vi "JKI_ErrorHandler.vi"() -> ()   [LabVIEW 2017, in "Error Handler_JKI.lvlib"]
uses:
  APIs/Error Handler_JKI.lvlib
  <userlib>/_NEVSTOP/JKI State Machine ++/_Support/_JKISMQFGV.vi
  <userlib>/_NEVSTOP/JKI State Machine ++/JKI-State-Machine-Plus.lvlib
panel:
  in  "Error Simulator":bool
  in  "Stop Button":bool
  out "State History":string
  in  "Name(\"\" to use uuid)":string="Event JKISM"
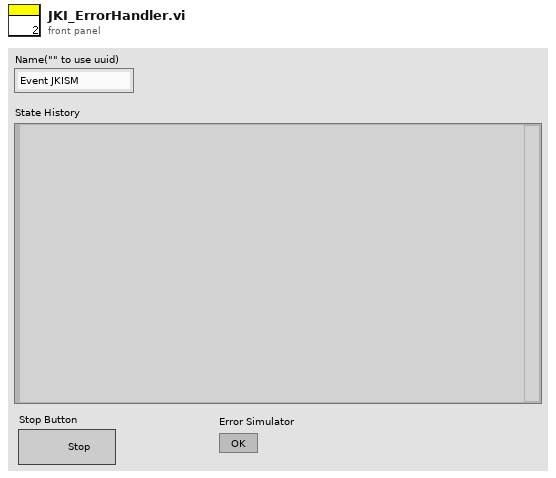
[diagram p1: front panel]
types:
  T1 = enum32{"Invalid", "Standard", "Closed", "Hidden", "Minimized", "Maximized"}
  T2 = enum32{"invalid app kind", "Development System", "Run Time System", "Student Edition", "Embedded LabVIEW", "Evaluation", "Custom"}
  T3 = enum16{"open", "replace", "create", "open or create", "replace or create", "replace or create with confirmation"}
  T4 = cluster{"Core":cluster{"Current VI Reference":refnum<vi>, "Close Panel on Exit?":bool}, "Your Boolean data":bool, "Your string data":string}
  T5 = cluster{"Current VI Reference":refnum<vi>, "Close Panel on Exit?":bool}
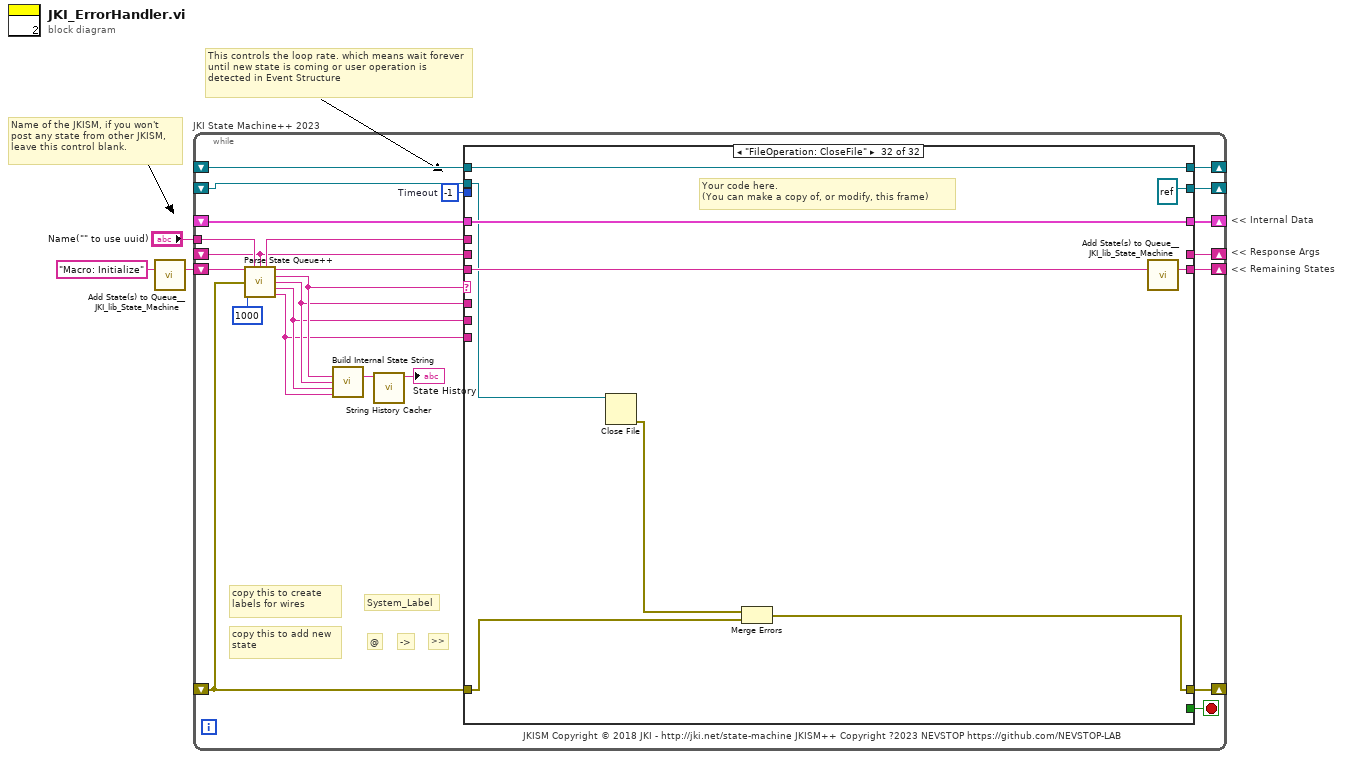
[diagram p0: block diagram]
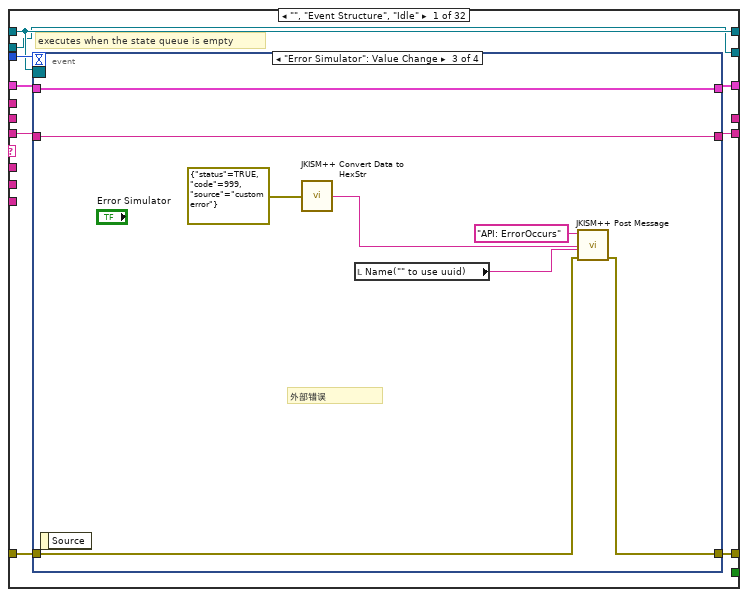
[diagram p2: hidden frame]
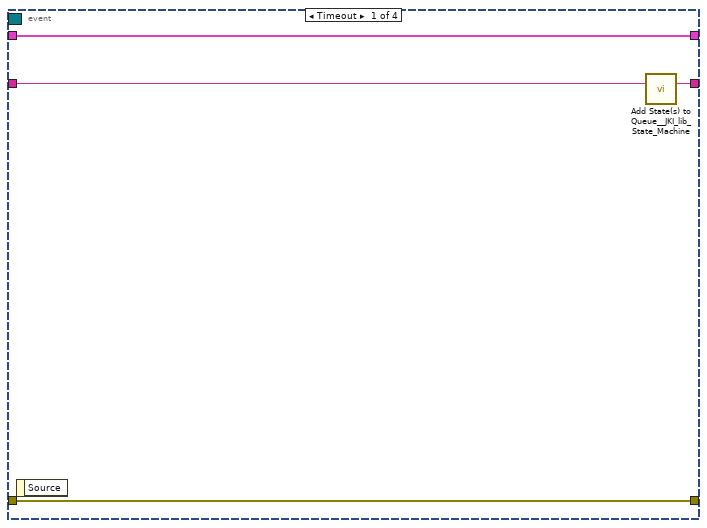
[diagram p3: hidden frame]
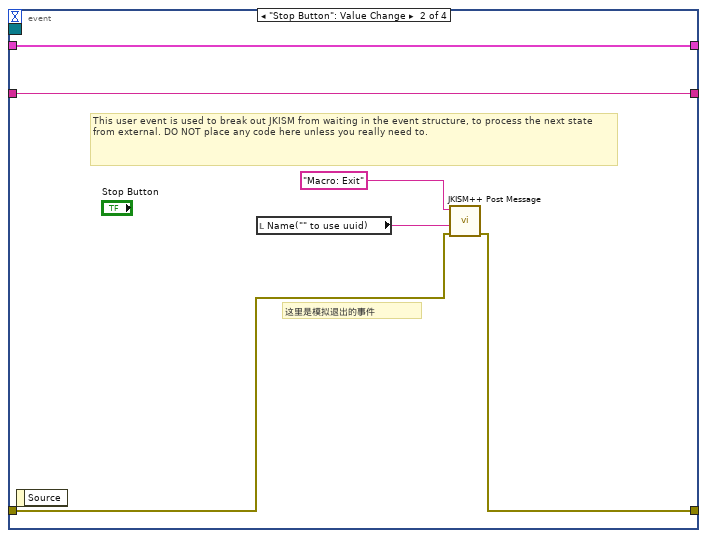
[diagram p4: hidden frame]
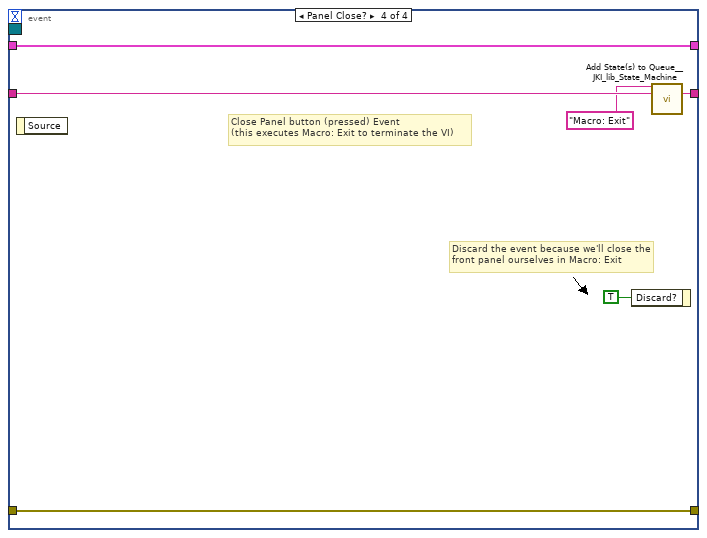
[diagram p5: hidden frame]
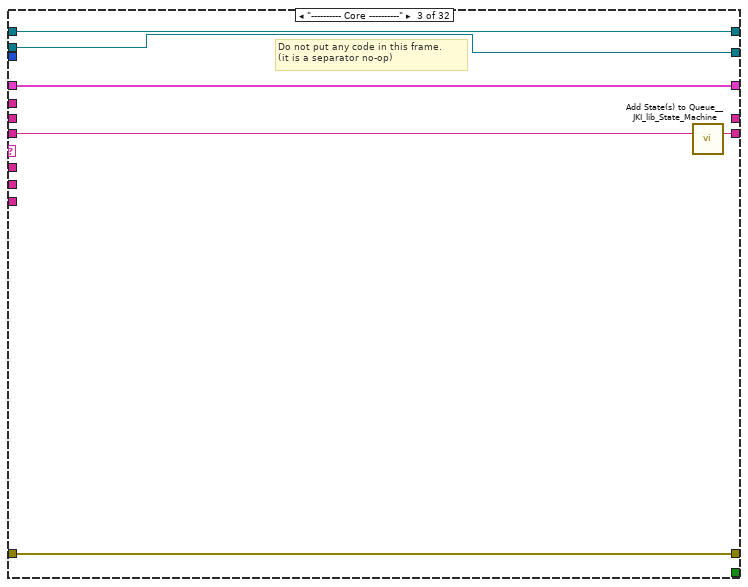
[diagram p7: hidden frame]
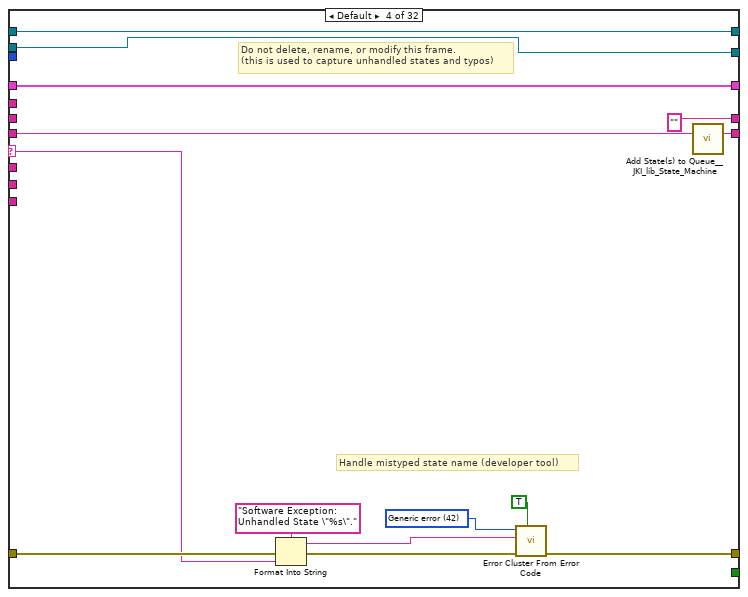
[diagram p8: hidden frame]
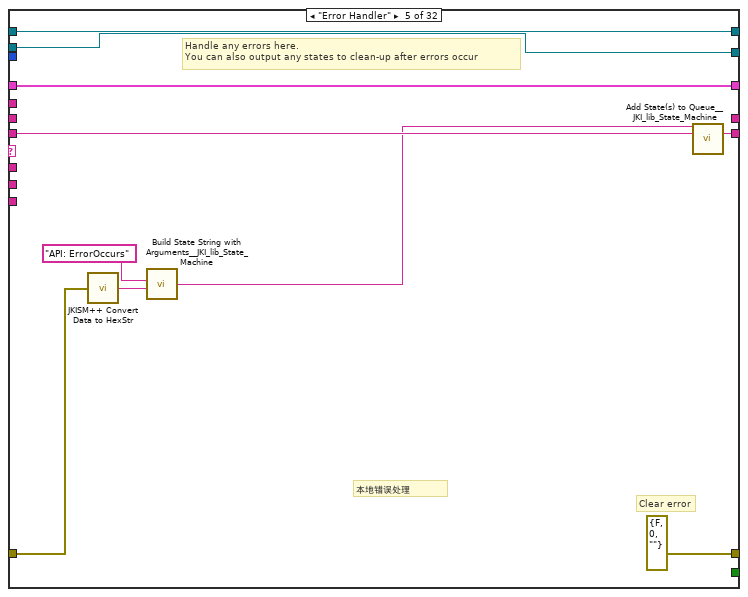
[diagram p9: hidden frame]
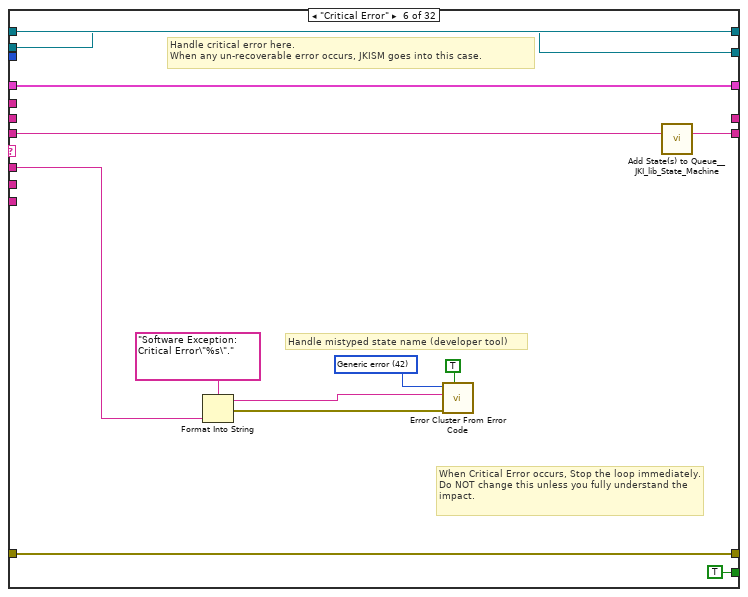
[diagram p10: hidden frame]
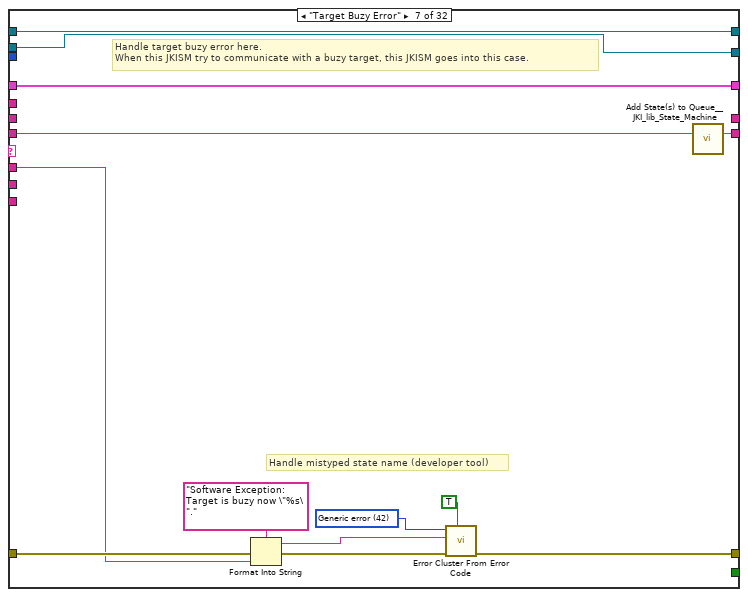
[diagram p11: hidden frame]
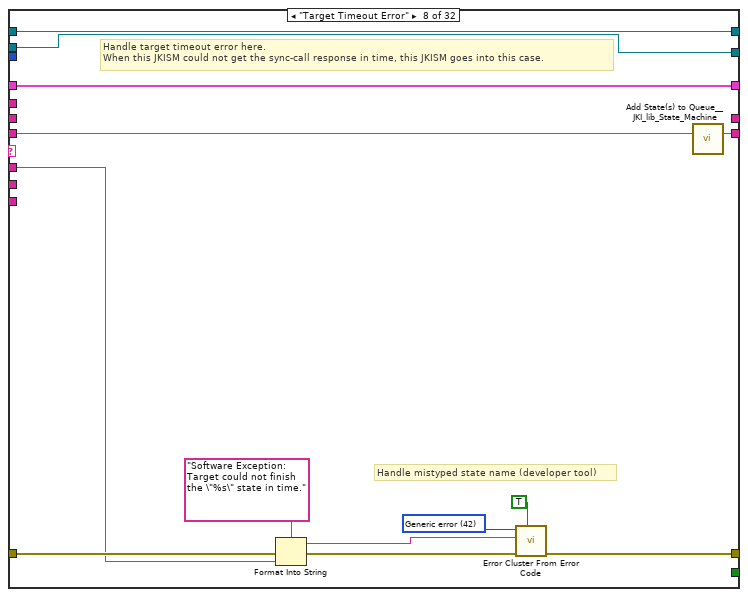
[diagram p12: hidden frame]
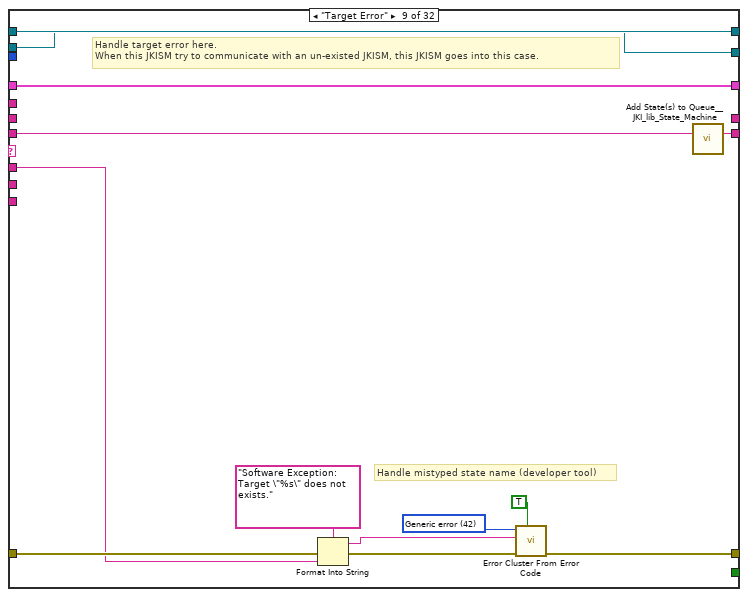
[diagram p13: hidden frame]
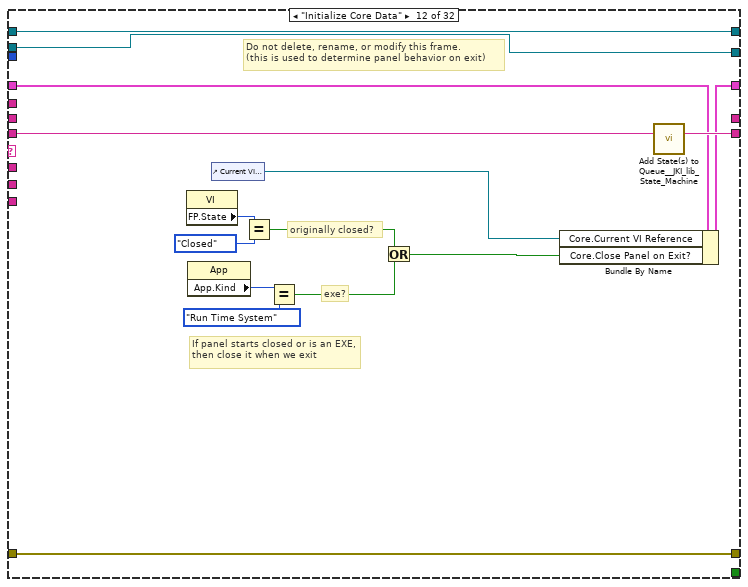
[diagram p16: hidden frame]
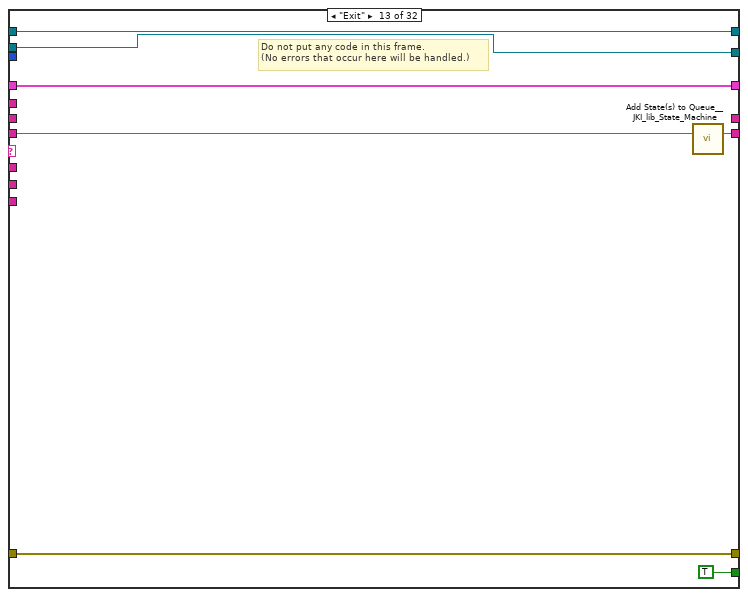
[diagram p17: hidden frame]
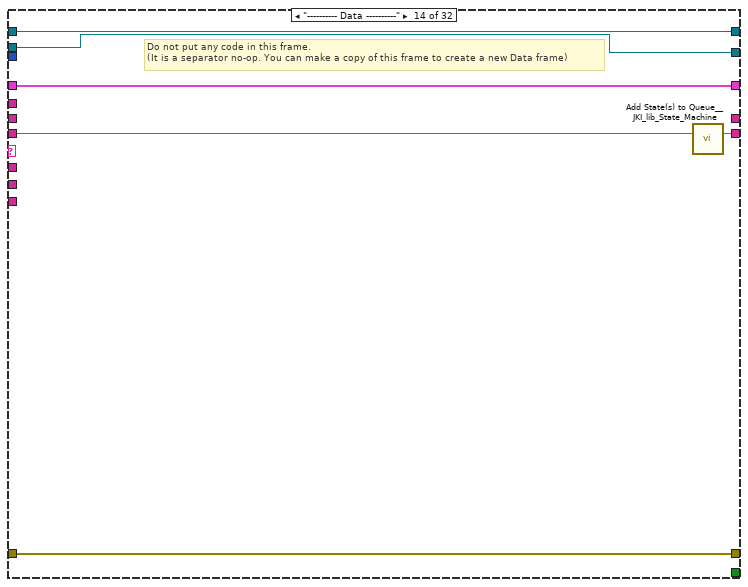
[diagram p18: hidden frame]
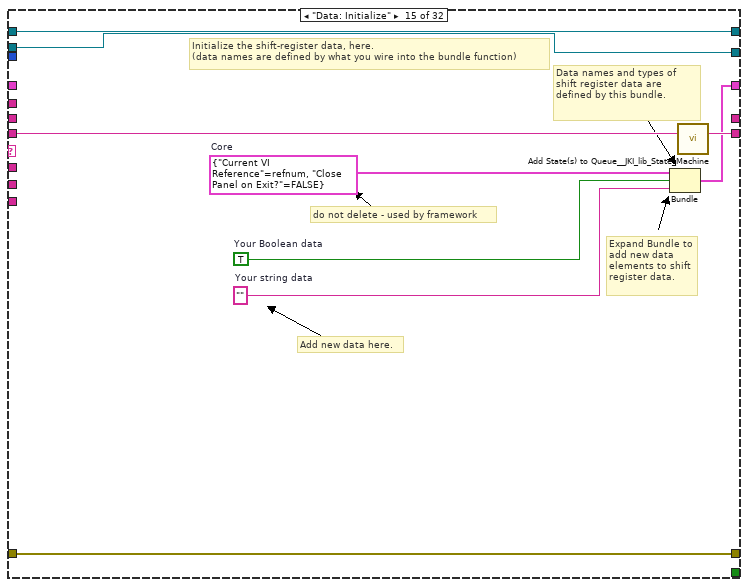
[diagram p19: hidden frame]
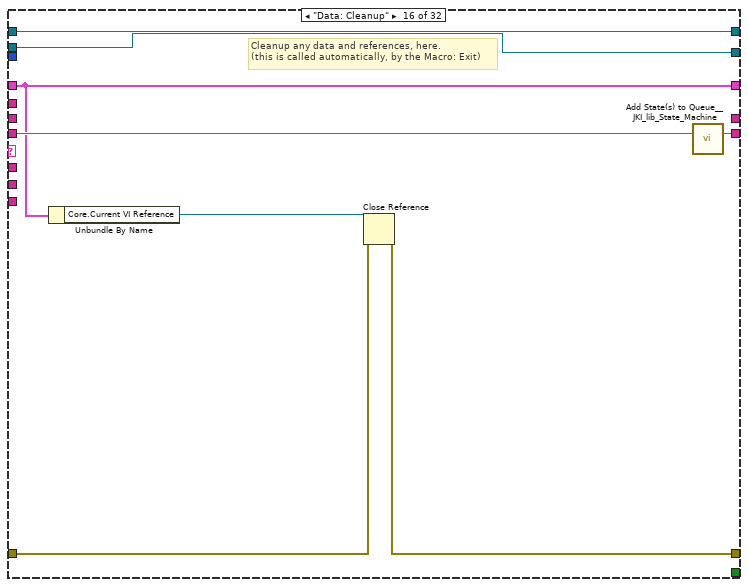
[diagram p20: hidden frame]
diagram:
  # "<< Internal Data"
  # "<< Response Args"
  # "<< Remaining States"
  # "Name of the JKISM, if you won't post any state from other JKISM,  leave this control blank."
  # "This controls the loop rate. which means wait forever until new state is coming or user operation is detected in Event Structure"
  n1 = call <vilib>:"Add State(s) to Queue__JKI_lib_State_Machine.vi"("State(s) in (\"\")"="Macro: Initialize") -> ("States Out"=w1:string)  [unwired: 14 in]
  n2 = while "JKI State Machine++ 2023" {
    shift-right: [w22] -> _
    shift-left: _ -> [w21]
    shift-right: [w25] -> _
    shift-left: _ -> [w19]
    shift-right: [w24] -> _
    shift-left: w1 -> [w26]
    tunnel: "Name(\"\" to use uuid)" -> [w14]
    shift-right: [w17] -> _
    shift-left: _ -> [w6]
    shift-right: [w16] -> _
    shift-left: _ -> [w15]
    shift-right: [w5] -> _
    shift-left: _ -> [w4]
    stop <- w23 stop-if-true
    w20 = -1  # Timeout
    # "JKISM Copyright © 2018 JKI - http://jki.net/state-machine JKISM++ Copyright ?2023 NEVSTOP https://github.com/NEVSTOP-LAB"
    # "copy this to add new state"
    # ">>"
    # "->"
    # "@"
    # "copy this to create labels for wires"
    # "System_Label"
    n3 = call <userlib>:"Parse State Queue++.vi"("State Queue"=w26, "Name(\"\" to use uuid)"=w14, "Response Arguments"=w6, "Error In (no error)"=w19, "Response Timeout(5000ms)"=1000 ("Response Timeout(1000ms)")) -> ("Name Used"=w7:string, "Remaining States"=w27:string, "Current State"=w11:string, "Arguments"=w10:string, "Argument - State"=w9:string, "From Who"=w8:string)  [unwired: 5 in]
    n4 = call <userlib>:"Build Internal State String.vi"("State"=w11, "Arguments (\"\")"=w10, "Arg-State (\"\")"=w9, "Source (\"\")"=w8) -> ("State with Arguments"=w12:string)  [unwired: 11 in]
    n5 = call <userlib>:"String History Cacher.vi"("String"=w12) -> ("String Cache"=→"State History":string)  [unwired: 10 in]
    n6 = case shown="\"FileOperation: CloseFile\"" w11 {
      selector: w11 -> [_ _ _ w75 _ _ _ _ _ _ _ _ _ _ _ _ _ _ _ _ _ _ _ _ _ _ _ _ _ _ _ _]
      tunnel: w27 -> [w36 w64 w71 w79 w95 w106 w110 w128 w141 w151 w156 w172 w179 w185 w194 w202 w208 w215 w220 w227 w233 w241 w254 w325 w332 w344 w348 w352 w374 w391 w400 w409]
      tunnel: w10 -> [_ _ _ _ _ w99 w112 w124 w137 _ _ _ _ _ _ _ _ _ _ _ _ w236 w248 _ _ _ _ w369 _ _ _ _]
      tunnel: w21 -> [w34 w63 w68 w77 w92 w107 w114 w126 w139 w150 w155 w165 w177 w182 _ w197 w205 w214 w219 w224 w231 w239 w250 w322 w329 w341 w347 w371 w380 w388 w398 w407]
      tunnel: [w33 w65 w69 w81 errorcluster {"status"=FALSE, "code"=0, "source"=""} ("error out") w108 w117 w130 w143 w152 w157 w169 w176 w183 w191 w198 w206 w210 w218 w225 w230 w237 w251 w323 w330 w342 w349 w354 w376 w389 w392 w401] -> w25
      tunnel: w19 -> [w32 w65 w69 w80 w89 w108 w116 w129 w142 w152 w157 w169 w176 w183 w191 w199 w206 _ w221 w225 w230 w238 w252 w323 w330 w342 w349 w366 w377 w389 w393 w403]
      tunnel: [w35 w64 w70 w78 w94 w105 w115 w127 w140 w151 w156 w171 w178 w184 w193 w201 w207 w215 w220 w226 w232 w240 w253 w324 w331 w343 w348 w351 w373 w390 w399 w408] -> w24
      tunnel: [_ _ _ _ _ TRUE _ _ _ _ _ _ TRUE _ _ _ _ _ _ _ _ _ _ _ _ _ _ _ TRUE _ _ _] -> w23
      tunnel: [w31 w63 w68 w77 w92 w107 w114 w126 w139 w150 w155 w170 w177 w182 w192 w197 w205 w214 w219 w224 w231 w239 w250 w322 w329 w341 w347 w371 w380 w388 w398 w407] -> w22
      tunnel: w20 -> [w30 _ _ _ _ _ _ _ _ _ _ _ _ _ _ _ _ _ _ _ _ _ _ _ _ _ _ _ _ _ _ _]
      tunnel: w8 -> [_ _ _ _ _ _ _ _ _ _ _ _ _ _ _ _ _ _ _ _ _ _ _ _ _ _ _ w362 _ _ _ _]
      tunnel: w9 -> [_ _ _ _ _ _ _ _ _ _ _ _ _ _ _ _ _ _ _ _ _ _ _ _ _ _ _ _ _ _ _ _]
      tunnel: [_ _ _ "" _ _ _ _ _ _ _ _ _ _ _ _ _ _ _ _ _ _ _ _ _ _ _ _ _ _ _ _] -> w17
      tunnel: [w29 w62 w67 w73 w91 w97 w111 w123 w136 w149 w154 w159 w174 w181 w187 w196 w204 w213 w217 w223 w229 w235 w247 w321 w327 w334 w346 w370 w379 w387 w397 w406] -> w16
      tunnel: w15 -> [w29 w62 w67 w73 w91 w97 w111 w123 w136 w149 w154 w159 w174 w181 w187 w196 w204 _ w217 w223 w229 w235 w247 w321 w327 w334 w346 w370 w379 w387 w397 w406]
      tunnel: w7 -> [_ _ _ _ _ _ _ _ _ _ _ _ _ _ _ _ _ w212 _ _ _ _ _ _ _ _ _ _ _ _ _ _]
      tunnel: w6 -> [_ _ _ _ _ _ _ _ _ _ _ _ _ _ _ _ _ _ _ _ _ _ _ _ _ _ _ _ _ _ _ _]
      tunnel: [w28 w61 w66 w72 w90 w96 w109 w122 w135 w148 w153 w158 w173 w180 w186 w195 w203 w209 w216 w222 w228 w234 w246 w320 w326 w333 w345 w353 w378 w386 w394 refnum<file> refnum ("refnum out")] -> w5
      tunnel: w4 -> [w28 w61 w66 w72 w90 w96 w109 w122 w135 w148 w153 w158 w173 w180 w186 w195 w203 w209 w216 w222 w228 w234 w246 w320 w326 w333 w345 w357 w378 w386 _ w405]
      frame "", "Event Structure", "Idle" {
        # "executes when the state queue is empty"
        n7 = event shown="[2] \"Error Simulator\": Value Change" {
          selector: w29 -> [_ _ _ _]
          dyn-events: _ -> [_ _ _ _]
          timeout: w30 -> [_ _ _ _]
          tunnel: w36 -> [w40 w45 w54 w60]
          tunnel: [w39 w45 w54 w59] -> w35
          tunnel: w34 -> [w37 w46 w53 w57]
          tunnel: [w38 w41 w47 w58] -> w33
          tunnel: w32 -> [w38 w42 w48 w58]
          tunnel: [w37 w46 w53 w57] -> w31
          event Timeout {
            n8 = event-data() -> ()  [unwired: 1 in, 1 out]
            n9 = call <vilib>:"Add State(s) to Queue__JKI_lib_State_Machine.vi"("State(s) in (\"\")"=w40) -> ("States Out"=w39:string)  [unwired: 14 in]
          }
          event "Stop Button": Value Change {
            # "这里是模拟退出的事件"
            # "This user event is used to break out JKISM from waiting in the event structure, to process the next state from external. DO NOT place any code here unless you really need to."
            n10 = event-data() -> ()  [unwired: 1 in, 1 out]
            n11 = local read "Name(\"\" to use uuid)"() -> (w44:string)
            n12 = call <userlib>:"JKISM++ Post Message.vi"("Error In (no error)"=w42, "Dest Module"=w44, "States"="Macro: Exit" ("Name(\"\" to use uuid)")) -> ("error IO"=w41:errorcluster)  [unwired: 8 in]
          }
          event "Error Simulator": Value Change {
            # "外部错误"
            n13 = event-data() -> ()  [unwired: 1 in, 1 out]
            n14 = call <userlib>:"JKISM++ Convert Data to HexStr.vi"("Variant"=errorcluster {"status"=TRUE, "code"=999, "source"="custom error"} ("error in (no error)")) -> ("HEX String (0-9,A-F)"=w49:string)  [unwired: 8 in]
            n15 = local read "Name(\"\" to use uuid)"() -> (w52:string)
            n16 = call <userlib>:"JKISM++ Post Message.vi"("Error In (no error)"=w48, "Dest Module"=w52, "Arguments (\"\")"=w49, "States"="API: ErrorOccurs") -> ("error IO"=w47:errorcluster)  [unwired: 7 in]
          }
          event Panel Close? {
            # "Discard the event because we'll close the front panel ourselves in Macro: Exit"
            # "Close Panel button (pressed) Event\n(this executes Macro: Exit to terminate the VI)"
            n17 = event-data() -> ()  [unwired: 1 in, 1 out]
            n18 = event-data("Discard?"=TRUE) -> ()  [unwired: 1 in, 1 out]
            n19 = call <vilib>:"Add State(s) to Queue__JKI_lib_State_Machine.vi"("State(s) in Front (\"\")"="Macro: Exit", "State(s) in (\"\")"=w60) -> ("States Out"=w59:string)  [unwired: 13 in]
          }
        }
      }
      frame "JKISM++ Documentation" {
        # "JKISM++ Documentation"
        # "State Syntax:\nStateCategory: State >> Argument @|-> JKISMName\nLine Terminator: Line feed\n\nExample:\nUI: Help >> About @Main\nUI: Help >> About ->Main"
        # "Commenting:\nTo add a comment use \"//\" or \"#\" and all text to the right will be ignored\nCommenting Example:\nUI: Initialize // This initializes the UI\n# This whole line is a comment\n// Another comment line"
        # "Where \"UI\" is the state category\nWhere \"Help\" is the state\nWhere \"About\" is the argument\nWhere \"Main\" is the Name of JKISM,which actually run the \"UI: Help >> About\"\n\n    \"@\" stands for sync state. Current JKISM will wait until the state is finished. \n            - if \"Main\" named JKISM does not exist, \"Target Error\" will occur.\n            - if \"Main\" named JKISM is in another sync remote state, \"Target Buzy Error\" will occur.\n            - if \"Main\" named JKISM could not finish the state in time, \"Target Timeout Error\" will occur.\n            - if everything is right. \"Response\" will occur with Argument back from \"Main\" named JKISM. \n\n    \"->\" stands for async state. Current JKISM will post the state and continue to next state in next iteration.\n            - if \"Main\" named JKISM does not exist, \"Target Error\" will occur.\n            - if everything is right. \"Async Message Posted\" will occur.\n            - After State is finished. Caller will receive a \"Async Response\" state from callee.\n\nWhen duplicated name is used for multiple JKISM module or some framework problem happens, \"Critical Error\" will occur."
      }
      frame "---------- Core ----------" {
        # "Do not put any code in this frame.\n(it is a separator no-op)"
        n20 = call <vilib>:"Add State(s) to Queue__JKI_lib_State_Machine.vi"("State(s) in (\"\")"=w71) -> ("States Out"=w70:string)  [unwired: 14 in]
      }
      frame Default {
        w84 = 42 items=["No error", "Argument error", "Memory is full", "Out of zone", "End of file", "File already open", "Generic file I/O error", "File not found", "File permission error", "Disk is full", "Duplicate path", "Too many files open", "System feature not enabled", "Resource file not found", "Cannot add resource", "Resource not found", "Image not found", "Image memory error", "Pen does not exist", "Config type invalid", "Config token not found", "Config parse error", "Config memory error", "Bad external code format", "Bad external code offset", "External code not present", "Null window", "Destroy window error", "Null menu", "Print aborted", "Bad print record", "Print driver error", "Windows error during printing", "Memory error during printing", "Print dialog error", "Generic print error", "Invalid device refnum", "Device not found", "Device parameter error", "Device unit error", "Cannot open device", "Device call aborted", "Generic error", "Cancelled by user", "Object ID too low", "Object ID too high", "Object not in heap", "Unknown heap", "Unknown object (invalid DefProc)", "Unknown object (DefProc not in table)", "Message out of range", "Invalid (null) method", "Unknown message", "Manager call not supported", "Bad address", "Network operation in progress", "Network operation timed out", "Connection is busy", "Network attribute not supported", "Network error", "Address in use", "System out of memory", "Connection aborted", "Connection refused", "Not connected", "Already connected", "Connection closed", "Initialization error (interapplication manager)", "Bad occurrence", "Wait on unbound occurrence handler", "Occurrence queue overflow", "Datalog type conflict", "Unused", "Unrecognized type (interapplication manager)", "Memory corrupt", "Failed to make temporary DLL", "Old CIN version", "Drag socket not found", "Failed to load drop-object", "Failed to register OLE object", "Failed to release OLE object", "Format specifier type mismatch", "Unknown format specifier", "Too few format specifiers", "Too many format specifiers", "Scan failed", "Newer CIN version", "Error converting to variant", "Runtime menu error", "Password tampered", "Variant attribute not found", "Incompatible variant data type", "Event data is not available", "Event Store is not present", "Occurrence is not found", "Event Queue is not created", "Event info is not available", "Refnum passed is NULL", "Error retrieving Class GUID", "Error retrieving CoClass GUID", "Error retrieving TypeLib GUID.", "Bad built application magic bytes.", "Specific driver is different from the specific driver associated with the Logical Name.", "There is no session opened to the class driver.", "Max Error", "MAX - Error with config objects", "MAX - Error loading configuration", "MAX - Group not supported"]
        # "Do not delete, rename, or modify this frame.\n(this is used to capture unhandled states and typos)"
        # "Handle mistyped state name (developer tool)"
        n21 = Format Into String(format string="Software Exception: Unhandled State \"%s\"." ("message"), error in=w80, w75) -> (resulting string=w83:string, error out=w82:errorcluster)  [unwired: 1 in]
        n22 = call <vilib>:"Error Cluster From Error Code.vi"("show call chain? (False)"=TRUE, "error in (no error)"=w82, "error message (\"\")"=w83, "error code (0)"=w84) -> ("error out"=w81:errorcluster)  [unwired: 5 in]
        n23 = call <vilib>:"Add State(s) to Queue__JKI_lib_State_Machine.vi"("State(s) in (\"\")"=w79) -> ("States Out"=w78:string)  [unwired: 14 in]
      }
      frame "Error Handler" {
        # "本地错误处理"
        # "Handle any errors here.\nYou can also output any states to clean-up after errors occur"
        # "Clear error"
        n24 = call <userlib>:"JKISM++ Convert Data to HexStr.vi"("Variant"=w89) -> ("HEX String (0-9,A-F)"=w88:string)  [unwired: 8 in]
        n25 = call <vilib>:"Build State String with Arguments__JKI_lib_State_Machine.vi"("Arguments (\"\")"=w88, "State"="API: ErrorOccurs") -> ("State with Arguments"=w86:string)  [unwired: 4 in]
        n26 = call <vilib>:"Add State(s) to Queue__JKI_lib_State_Machine.vi"("State(s) in Front (\"\")"=w86, "State(s) in (\"\")"=w95) -> ("States Out"=w94:string)  [unwired: 13 in]
      }
      frame "Critical Error" {
        w103 = 42 items=["No error", "Argument error", "Memory is full", "Out of zone", "End of file", "File already open", "Generic file I/O error", "File not found", "File permission error", "Disk is full", "Duplicate path", "Too many files open", "System feature not enabled", "Resource file not found", "Cannot add resource", "Resource not found", "Image not found", "Image memory error", "Pen does not exist", "Config type invalid", "Config token not found", "Config parse error", "Config memory error", "Bad external code format", "Bad external code offset", "External code not present", "Null window", "Destroy window error", "Null menu", "Print aborted", "Bad print record", "Print driver error", "Windows error during printing", "Memory error during printing", "Print dialog error", "Generic print error", "Invalid device refnum", "Device not found", "Device parameter error", "Device unit error", "Cannot open device", "Device call aborted", "Generic error", "Cancelled by user", "Object ID too low", "Object ID too high", "Object not in heap", "Unknown heap", "Unknown object (invalid DefProc)", "Unknown object (DefProc not in table)", "Message out of range", "Invalid (null) method", "Unknown message", "Manager call not supported", "Bad address", "Network operation in progress", "Network operation timed out", "Connection is busy", "Network attribute not supported", "Network error", "Address in use", "System out of memory", "Connection aborted", "Connection refused", "Not connected", "Already connected", "Connection closed", "Initialization error (interapplication manager)", "Bad occurrence", "Wait on unbound occurrence handler", "Occurrence queue overflow", "Datalog type conflict", "Unused", "Unrecognized type (interapplication manager)", "Memory corrupt", "Failed to make temporary DLL", "Old CIN version", "Drag socket not found", "Failed to load drop-object", "Failed to register OLE object", "Failed to release OLE object", "Format specifier type mismatch", "Unknown format specifier", "Too few format specifiers", "Too many format specifiers", "Scan failed", "Newer CIN version", "Error converting to variant", "Runtime menu error", "Password tampered", "Variant attribute not found", "Incompatible variant data type", "Event data is not available", "Event Store is not present", "Occurrence is not found", "Event Queue is not created", "Event info is not available", "Refnum passed is NULL", "Error retrieving Class GUID", "Error retrieving CoClass GUID", "Error retrieving TypeLib GUID.", "Bad built application magic bytes.", "Specific driver is different from the specific driver associated with the Logical Name.", "There is no session opened to the class driver.", "Max Error", "MAX - Error with config objects", "MAX - Error loading configuration", "MAX - Group not supported"]
        # "Handle critical error here.\nWhen any un-recoverable error occurs, JKISM goes into this case."
        # "When Critical Error occurs, Stop the loop immediately. Do NOT change this unless you fully understand the impact."
        # "Handle mistyped state name (developer tool)"
        n27 = Format Into String(format string="Software Exception: Critical Error\"%s\"." ("message"), w99) -> (resulting string=w102:string, error out=w101:errorcluster)  [unwired: 2 in]
        n28 = call <vilib>:"Error Cluster From Error Code.vi"("show call chain? (False)"=TRUE, "error in (no error)"=w101, "error message (\"\")"=w102, "error code (0)"=w103) -> ()  [unwired: 5 in, 1 out]
        n29 = call <vilib>:"Add State(s) to Queue__JKI_lib_State_Machine.vi"("State(s) in (\"\")"=w106) -> ("States Out"=w105:string)  [unwired: 14 in]
      }
      frame "Target Buzy Error" {
        w120 = 42 items=["No error", "Argument error", "Memory is full", "Out of zone", "End of file", "File already open", "Generic file I/O error", "File not found", "File permission error", "Disk is full", "Duplicate path", "Too many files open", "System feature not enabled", "Resource file not found", "Cannot add resource", "Resource not found", "Image not found", "Image memory error", "Pen does not exist", "Config type invalid", "Config token not found", "Config parse error", "Config memory error", "Bad external code format", "Bad external code offset", "External code not present", "Null window", "Destroy window error", "Null menu", "Print aborted", "Bad print record", "Print driver error", "Windows error during printing", "Memory error during printing", "Print dialog error", "Generic print error", "Invalid device refnum", "Device not found", "Device parameter error", "Device unit error", "Cannot open device", "Device call aborted", "Generic error", "Cancelled by user", "Object ID too low", "Object ID too high", "Object not in heap", "Unknown heap", "Unknown object (invalid DefProc)", "Unknown object (DefProc not in table)", "Message out of range", "Invalid (null) method", "Unknown message", "Manager call not supported", "Bad address", "Network operation in progress", "Network operation timed out", "Connection is busy", "Network attribute not supported", "Network error", "Address in use", "System out of memory", "Connection aborted", "Connection refused", "Not connected", "Already connected", "Connection closed", "Initialization error (interapplication manager)", "Bad occurrence", "Wait on unbound occurrence handler", "Occurrence queue overflow", "Datalog type conflict", "Unused", "Unrecognized type (interapplication manager)", "Memory corrupt", "Failed to make temporary DLL", "Old CIN version", "Drag socket not found", "Failed to load drop-object", "Failed to register OLE object", "Failed to release OLE object", "Format specifier type mismatch", "Unknown format specifier", "Too few format specifiers", "Too many format specifiers", "Scan failed", "Newer CIN version", "Error converting to variant", "Runtime menu error", "Password tampered", "Variant attribute not found", "Incompatible variant data type", "Event data is not available", "Event Store is not present", "Occurrence is not found", "Event Queue is not created", "Event info is not available", "Refnum passed is NULL", "Error retrieving Class GUID", "Error retrieving CoClass GUID", "Error retrieving TypeLib GUID.", "Bad built application magic bytes.", "Specific driver is different from the specific driver associated with the Logical Name.", "There is no session opened to the class driver.", "Max Error", "MAX - Error with config objects", "MAX - Error loading configuration", "MAX - Group not supported"]
        # "Handle target buzy error here.\nWhen this JKISM try to communicate with a buzy target, this JKISM goes into this case."
        # "Handle mistyped state name (developer tool)"
        n30 = Format Into String(format string="Software Exception: Target is buzy now \"%s\"." ("message"), error in=w116, w112) -> (resulting string=w119:string, error out=w118:errorcluster)  [unwired: 1 in]
        n31 = call <vilib>:"Error Cluster From Error Code.vi"("show call chain? (False)"=TRUE, "error in (no error)"=w118, "error message (\"\")"=w119, "error code (0)"=w120) -> ("error out"=w117:errorcluster)  [unwired: 5 in]
        n32 = call <vilib>:"Add State(s) to Queue__JKI_lib_State_Machine.vi"("State(s) in (\"\")"=w110) -> ("States Out"=w115:string)  [unwired: 14 in]
      }
      frame "Target Timeout Error" {
        w133 = 42 items=["No error", "Argument error", "Memory is full", "Out of zone", "End of file", "File already open", "Generic file I/O error", "File not found", "File permission error", "Disk is full", "Duplicate path", "Too many files open", "System feature not enabled", "Resource file not found", "Cannot add resource", "Resource not found", "Image not found", "Image memory error", "Pen does not exist", "Config type invalid", "Config token not found", "Config parse error", "Config memory error", "Bad external code format", "Bad external code offset", "External code not present", "Null window", "Destroy window error", "Null menu", "Print aborted", "Bad print record", "Print driver error", "Windows error during printing", "Memory error during printing", "Print dialog error", "Generic print error", "Invalid device refnum", "Device not found", "Device parameter error", "Device unit error", "Cannot open device", "Device call aborted", "Generic error", "Cancelled by user", "Object ID too low", "Object ID too high", "Object not in heap", "Unknown heap", "Unknown object (invalid DefProc)", "Unknown object (DefProc not in table)", "Message out of range", "Invalid (null) method", "Unknown message", "Manager call not supported", "Bad address", "Network operation in progress", "Network operation timed out", "Connection is busy", "Network attribute not supported", "Network error", "Address in use", "System out of memory", "Connection aborted", "Connection refused", "Not connected", "Already connected", "Connection closed", "Initialization error (interapplication manager)", "Bad occurrence", "Wait on unbound occurrence handler", "Occurrence queue overflow", "Datalog type conflict", "Unused", "Unrecognized type (interapplication manager)", "Memory corrupt", "Failed to make temporary DLL", "Old CIN version", "Drag socket not found", "Failed to load drop-object", "Failed to register OLE object", "Failed to release OLE object", "Format specifier type mismatch", "Unknown format specifier", "Too few format specifiers", "Too many format specifiers", "Scan failed", "Newer CIN version", "Error converting to variant", "Runtime menu error", "Password tampered", "Variant attribute not found", "Incompatible variant data type", "Event data is not available", "Event Store is not present", "Occurrence is not found", "Event Queue is not created", "Event info is not available", "Refnum passed is NULL", "Error retrieving Class GUID", "Error retrieving CoClass GUID", "Error retrieving TypeLib GUID.", "Bad built application magic bytes.", "Specific driver is different from the specific driver associated with the Logical Name.", "There is no session opened to the class driver.", "Max Error", "MAX - Error with config objects", "MAX - Error loading configuration", "MAX - Group not supported"]
        # "Handle target timeout error here.\nWhen this JKISM could not get the sync-call response in time, this JKISM goes into this case."
        # "Handle mistyped state name (developer tool)"
        n33 = Format Into String(format string="Software Exception: Target could not finish the \"%s\" state in time." ("message"), error in=w129, w124) -> (resulting string=w132:string, error out=w131:errorcluster)  [unwired: 1 in]
        n34 = call <vilib>:"Error Cluster From Error Code.vi"("show call chain? (False)"=TRUE, "error in (no error)"=w131, "error message (\"\")"=w132, "error code (0)"=w133) -> ("error out"=w130:errorcluster)  [unwired: 5 in]
        n35 = call <vilib>:"Add State(s) to Queue__JKI_lib_State_Machine.vi"("State(s) in (\"\")"=w128) -> ("States Out"=w127:string)  [unwired: 14 in]
      }
      frame "Target Error" {
        w146 = 42 items=["No error", "Argument error", "Memory is full", "Out of zone", "End of file", "File already open", "Generic file I/O error", "File not found", "File permission error", "Disk is full", "Duplicate path", "Too many files open", "System feature not enabled", "Resource file not found", "Cannot add resource", "Resource not found", "Image not found", "Image memory error", "Pen does not exist", "Config type invalid", "Config token not found", "Config parse error", "Config memory error", "Bad external code format", "Bad external code offset", "External code not present", "Null window", "Destroy window error", "Null menu", "Print aborted", "Bad print record", "Print driver error", "Windows error during printing", "Memory error during printing", "Print dialog error", "Generic print error", "Invalid device refnum", "Device not found", "Device parameter error", "Device unit error", "Cannot open device", "Device call aborted", "Generic error", "Cancelled by user", "Object ID too low", "Object ID too high", "Object not in heap", "Unknown heap", "Unknown object (invalid DefProc)", "Unknown object (DefProc not in table)", "Message out of range", "Invalid (null) method", "Unknown message", "Manager call not supported", "Bad address", "Network operation in progress", "Network operation timed out", "Connection is busy", "Network attribute not supported", "Network error", "Address in use", "System out of memory", "Connection aborted", "Connection refused", "Not connected", "Already connected", "Connection closed", "Initialization error (interapplication manager)", "Bad occurrence", "Wait on unbound occurrence handler", "Occurrence queue overflow", "Datalog type conflict", "Unused", "Unrecognized type (interapplication manager)", "Memory corrupt", "Failed to make temporary DLL", "Old CIN version", "Drag socket not found", "Failed to load drop-object", "Failed to register OLE object", "Failed to release OLE object", "Format specifier type mismatch", "Unknown format specifier", "Too few format specifiers", "Too many format specifiers", "Scan failed", "Newer CIN version", "Error converting to variant", "Runtime menu error", "Password tampered", "Variant attribute not found", "Incompatible variant data type", "Event data is not available", "Event Store is not present", "Occurrence is not found", "Event Queue is not created", "Event info is not available", "Refnum passed is NULL", "Error retrieving Class GUID", "Error retrieving CoClass GUID", "Error retrieving TypeLib GUID.", "Bad built application magic bytes.", "Specific driver is different from the specific driver associated with the Logical Name.", "There is no session opened to the class driver.", "Max Error", "MAX - Error with config objects", "MAX - Error loading configuration", "MAX - Group not supported"]
        # "Handle target error here.\nWhen this JKISM try to communicate with an un-existed JKISM, this JKISM goes into this case."
        # "Handle mistyped state name (developer tool)"
        n36 = Format Into String(format string="Software Exception: Target \"%s\" does not exists." ("message"), error in=w142, w137) -> (resulting string=w145:string, error out=w144:errorcluster)  [unwired: 1 in]
        n37 = call <vilib>:"Error Cluster From Error Code.vi"("show call chain? (False)"=TRUE, "error in (no error)"=w144, "error message (\"\")"=w145, "error code (0)"=w146) -> ("error out"=w143:errorcluster)  [unwired: 5 in]
        n38 = call <vilib>:"Add State(s) to Queue__JKI_lib_State_Machine.vi"("State(s) in (\"\")"=w141) -> ("States Out"=w140:string)  [unwired: 14 in]
      }
      frame "Async Response", "Response" {
        # "Handle Async-call Response (\"Async Response\" for ->)"
        # "Handle Sync-call Response (\"Response\" for @)"
        # "After Message is excuted, JKISM+ goes to this state for recieve the response. \n    For Async Message(->), \"Async Response\" is used. This JKISM will goes to \"Async Message Posted\" immediately and recieve the \"Async Response\" after the callee finishes the message.\n    For Sync Message(@),  This JKISM will wait until the message is done and immidieatly goes to \"Response\""
      }
      frame "Async Message Posted" {
        # "Handle post action for async message (->)."
        # "After Async Message is posted (->), JKISM+ goes to this state for post-action. You can use Argument - State to tell which Async Message is called."
      }
      frame "Initialize Core Data" {
        # "Do not delete, rename, or modify this frame.\n(this is used to determine panel behavior on exit)"
        # "originally closed?"
        # "exe?"
        # "If panel starts closed or is an EXE, then close it when we exit"
        n39 = property class="VI"() -> ("FP.State"=w162:T1)  [unwired: 2 in, 2 out]
        n40 = property class="App"() -> ("App.Kind"=w168:T2)  [unwired: 2 in, 2 out]
        n41 = control-ref of="Current VI Reference"() -> (w163:refnum<vi>)
        n42 = Equal?(x=w162, y=T1."Closed" ("Front Panel Window:State")) -> (x = y?=w160:bool)
        n43 = Equal?(x=w168, y=T2."Run Time System" ("Application:Kind")) -> (x = y?=w166:bool)
        n44 = Or(x=w160, y=w166) -> (x .or. y?=w164:bool)
        n45 = Bundle By Name(cluster=w165, "Core.Current VI Reference"=w163, "Core.Close Panel on Exit?"=w164) -> (w170:T4)
        n46 = call <vilib>:"Add State(s) to Queue__JKI_lib_State_Machine.vi"("State(s) in (\"\")"=w172) -> ("States Out"=w171:string)  [unwired: 14 in]
      }
      frame "Exit" {
        # "Do not put any code in this frame.\n(No errors that occur here will be handled.)"
        n47 = call <vilib>:"Add State(s) to Queue__JKI_lib_State_Machine.vi"("State(s) in (\"\")"=w179) -> ("States Out"=w178:string)  [unwired: 14 in]
      }
      frame "---------- Data ----------" {
        # "Do not put any code in this frame.\n(It is a separator no-op. You can make a copy of this frame to create a new Data frame)"
        n48 = call <vilib>:"Add State(s) to Queue__JKI_lib_State_Machine.vi"("State(s) in (\"\")"=w185) -> ("States Out"=w184:string)  [unwired: 14 in]
      }
      frame "Data: Initialize" {
        w188 = T5 {"Current VI Reference"=refnum, "Close Panel on Exit?"=FALSE}  # Core
        w190 = TRUE  # Your Boolean data
        w189 = ""  # Your string data
        # "do not delete - used by framework"
        # "Expand Bundle to add new data elements to shift register data."
        # "Add new data here."
        # "Data names and types of shift register data are defined by this bundle."
        # "Initialize the shift-register data, here.\n(data names are defined by what you wire into the bundle function)"
        n49 = Bundle("Core"=w188, "Your Boolean data"=w190, "Your string data"=w189) -> (w192:T4)  [unwired: 1 in]
        n50 = call <vilib>:"Add State(s) to Queue__JKI_lib_State_Machine.vi"("State(s) in (\"\")"=w194) -> ("States Out"=w193:string)  [unwired: 14 in]
      }
      frame "Data: Cleanup" {
        # "Cleanup any data and references, here.\n(this is called automatically, by the Macro: Exit)"
        n51 = Unbundle By Name(w197) -> ("Core.Current VI Reference"=w200:refnum<vi>)
        n52 = Close Reference(reference=w200, error in (no error)=w199) -> (error out=w198:errorcluster)
        n53 = call <vilib>:"Add State(s) to Queue__JKI_lib_State_Machine.vi"("State(s) in (\"\")"=w202) -> ("States Out"=w201:string)  [unwired: 14 in]
      }
      frame "---------- Events ----------" {
        # "Do not put any code in this frame.\n(It is a separator no-op. You can make a copy of this frame to create a new UI frame)"
        n54 = call <vilib>:"Add State(s) to Queue__JKI_lib_State_Machine.vi"("State(s) in (\"\")"=w208) -> ("States Out"=w207:string)  [unwired: 14 in]
      }
      frame "Events: Register" {
        # "Register message event to break Waiting in Event structure."
        n55 = call <userlib>:"JKISM++ Get New State Notifier Event.vi"("Name(\"\" to use uuid) in"=w212) -> ("Error out"=w210:errorcluster, "New State Notifier Event"=w211:refnum<user-event>)  [unwired: 9 in]
        n56 = register-events(w211) -> (reference out=w213:refnum<event-registration>)  [unwired: 2 in, 1 out]
      }
      frame "Events: Unregister" {
        n57 = Unregister For Events(event registration refnum=w217, error in=w221) -> (error out=w218:errorcluster)
      }
      frame "---------- UI ----------" {
        # "Do not put any code in this frame.\n(It is a separator no-op. You can make a copy of this frame to create a new UI frame)"
        n58 = call <vilib>:"Add State(s) to Queue__JKI_lib_State_Machine.vi"("State(s) in (\"\")"=w227) -> ("States Out"=w226:string)  [unwired: 14 in]
      }
      frame "UI: Initialize" {
        # "Initialize the User Interface, here.\n(this is called automatically, by the Macro: Init)"
        n59 = call <vilib>:"Add State(s) to Queue__JKI_lib_State_Machine.vi"("State(s) in (\"\")"=w233) -> ("States Out"=w232:string)  [unwired: 14 in]
      }
      frame "UI: Cursor Set" {
        # "Argument"
        # "Set and Unset Cursor Busy.\n(Usage: \"UI: Cursor Set >> Busy|Idle\")"
        n60 = case shown="\"Idle\", Default" w236 {
          tunnel: w238 -> [w243 w245]
          tunnel: [w242 w244] -> w237
          frame "Idle", Default {
            n61 = call <vilib>:"Unset Busy.vi"("error in (no error)"=w243) -> ("error out"=w242:errorcluster)  [unwired: 10 in]
          }
          frame "Busy" {
            n62 = call <vilib>:"Set Busy.vi"("error in (no error)"=w245) -> ("error out"=w244:errorcluster)  [unwired: 9 in, 1 out]
          }
        }
        n63 = call <vilib>:"Add State(s) to Queue__JKI_lib_State_Machine.vi"("State(s) in (\"\")"=w241) -> ("States Out"=w240:string)  [unwired: 14 in]
      }
      frame "UI: Front Panel State" {
        # "Argument"
        # "Set Front Panel Open or Closed\n(Usage: \"UI: Front Panel State >> Open|Close\")"
        n64 = Unbundle By Name(w250) -> ("Core.Current VI Reference"=w249:refnum<vi>)
        n65 = case shown="\"Minimize\", \"Minimized\"" w248 {
          tunnel: w252 -> [w260 w275 w286 w299 w312]
          tunnel: [w262 w276 w288 w301 w314] -> w251
          tunnel: w249 -> [w261 w273 w287 w300 w313]
          frame "Open", "Standard", Default {
            w255 = T1."Standard" ("State")
            n66 = property class="VI"(reference=w261, error in=w260) -> (reference out=w258:refnum<vi>, error out=w259:errorcluster, "FP.State"=w257:T1)
            n67 = Not Equal?(x=w257, y=w255) -> (x != y?=w256:bool)
            n68 = case shown="True" w256 {
              tunnel: [w266 w268] -> w262
              tunnel: w259 -> [w265 w268]
              tunnel: w258 -> [w264 _]
              tunnel: w255 -> [w263 _]
              frame True {
                n69 = invoke class="VI" method="FP.Open"(reference=w264, error in=w265, "Activate"=TRUE, "State"=w263) -> (error out=w266:errorcluster)  [unwired: 1 in, 4 out]
              }
              frame False {
              }
            }
          }
          frame "Close", "Closed" {
            n70 = property class="VI"(reference=w273, error in=w275) -> (reference out=w272:refnum<vi>, error out=w274:errorcluster, "FP.State"=w270:T1)
            n71 = Not Equal?(x=w270, y=T1."Closed" ("Front Panel Window:State")) -> (x != y?=w269:bool)
            n72 = case shown="True" w269 {
              tunnel: [w277 w280] -> w276
              tunnel: w274 -> [w277 w279]
              tunnel: w272 -> [_ w278]
              frame False {
              }
              frame True {
                n73 = invoke class="VI" method="FP.Close"(reference=w278, error in=w279) -> (error out=w280:errorcluster)  [unwired: 1 in, 2 out]
              }
            }
          }
          frame "Hidden", "Hide" {
            w281 = T1."Hidden" ("State")
            n74 = property class="VI"(reference=w287, error in=w286) -> (reference out=w284:refnum<vi>, error out=w285:errorcluster, "FP.State"=w283:T1)
            n75 = Not Equal?(x=w283, y=w281) -> (x != y?=w282:bool)
            n76 = case shown="True" w282 {
              tunnel: [w292 w293] -> w288
              tunnel: w285 -> [w291 w293]
              tunnel: w284 -> [w290 _]
              tunnel: w281 -> [w289 _]
              frame True {
                n77 = invoke class="VI" method="FP.Open"(reference=w290, error in=w291, "State"=w289) -> (error out=w292:errorcluster)  [unwired: 2 in, 4 out]
              }
              frame False {
              }
            }
          }
          frame "Minimize", "Minimized" {
            w294 = T1."Minimized" ("State")
            n78 = property class="VI"(reference=w300, error in=w299) -> (reference out=w297:refnum<vi>, error out=w298:errorcluster, "FP.State"=w296:T1)
            n79 = Not Equal?(x=w296, y=w294) -> (x != y?=w295:bool)
            n80 = case shown="True" w295 {
              tunnel: [w305 w306] -> w301
              tunnel: w298 -> [w304 w306]
              tunnel: w297 -> [w303 _]
              tunnel: w294 -> [w302 _]
              frame True {
                n81 = invoke class="VI" method="FP.Open"(reference=w303, error in=w304, "State"=w302) -> (error out=w305:errorcluster)  [unwired: 2 in, 4 out]
              }
              frame False {
              }
            }
          }
          frame "Maximize", "Maximized" {
            w307 = T1."Maximized" ("State")
            n82 = property class="VI"(reference=w313, error in=w312) -> (reference out=w310:refnum<vi>, error out=w311:errorcluster, "FP.State"=w309:T1)
            n83 = Not Equal?(x=w309, y=w307) -> (x != y?=w308:bool)
            n84 = case shown="True" w308 {
              tunnel: [w318 w319] -> w314
              tunnel: w311 -> [w317 w319]
              tunnel: w310 -> [w316 _]
              tunnel: w307 -> [w315 _]
              frame True {
                n85 = invoke class="VI" method="FP.Open"(reference=w316, error in=w317, "State"=w315) -> (error out=w318:errorcluster)  [unwired: 2 in, 4 out]
              }
              frame False {
              }
            }
          }
        }
        n86 = call <vilib>:"Add State(s) to Queue__JKI_lib_State_Machine.vi"("State(s) in (\"\")"=w254) -> ("States Out"=w253:string)  [unwired: 14 in]
      }
      frame "---------- Macro ----------" {
        # "Do not put any code in this frame.\n(It is a separator no-op. You can make a copy of this frame to create a new Macro frame)"
        n87 = call <vilib>:"Add State(s) to Queue__JKI_lib_State_Machine.vi"("State(s) in (\"\")"=w325) -> ("States Out"=w324:string)  [unwired: 14 in]
      }
      frame "Macro: Initialize" {
        w328 = "Data: Initialize\nInitialize Core Data\nEvents: Register\nUI: Initialize\nUI: Front Panel State >> Open\nFileOperation: OpenFile"  # Data: Initialize Initialize Core Data Events: Register UI: Initialize UI: Front Panel State >> Open FileOperation: OpenFile
        # "Initialization Macro\n(This is called once, when the VI starts)"
        n88 = call <vilib>:"Add State(s) to Queue__JKI_lib_State_Machine.vi"("State(s) in Front (\"\")"=w328, "State(s) in (\"\")"=w332) -> ("States Out"=w331:string)  [unwired: 13 in]
      }
      frame "Macro: Exit" {
        # "Exit Macro\n(This is called once, when the VI exits)"
        n89 = Unbundle By Name(w341) -> ("Core.Close Panel on Exit?"=w340:bool)
        n90 = Select(t="UI: Front Panel State >> Close", s=w340, f="") -> (s? t:f=w337:string)
        n91 = call <vilib>:"Add State(s) to Queue__JKI_lib_State_Machine.vi"("State(s) in (\"\")"=w337, "State(s) at Back (\"\")"="FileOperation: CloseFile\nData: Cleanup\nEvents: Unregister\nExit") -> ("States Out"=w335:string)  [unwired: 13 in]
        n92 = call <vilib>:"Add State(s) to Queue__JKI_lib_State_Machine.vi"("State(s) in Front (\"\")"=w335, "State(s) in (\"\")"=w344) -> ("States Out"=w343:string)  [unwired: 13 in]
      }
      frame "---------- API ----------" {
        # "Do not put any code in this frame.\n(It is a separator no-op. This category is recommanded to use for external API)"
      }
      frame "API: ErrorOccurs" {
        # "外部发送的error 接口\n系统中各个模块发生的错误信息处理，将时间+模块信息+错误编号+错误提示作为错误信息字符串。"
        # "unpack HexStr  to Variant\nif complex parameter is needed."
        # "Copy/Rename this case for your own API"
        n93 = call <userlib>:"JKISM++ Convert HexStr to Data.vi"("HEX String"=w369) -> ("Variant"=w368:variant)  [unwired: 8 in]
        n94 = Variant To Data(error in=w366, type=errorcluster {"status"=FALSE, "code"=0, "source"=""} ("error constant"), Variant=w368) -> (data=w365:errorcluster, error out=w358:errorcluster)
        n95 = Get Date/Time In Seconds() -> (seconds since 1Jan1904=w364:timestamp)
        n96 = Unbundle By Name(w365) -> ("code"=w361:i32, "source"=w360:string)
        n97 = Format Date/Time String(seconds (now)=w364) -> (date/time string=w363:string)  [unwired: 2 out]
        n98 = Format Into String(format string="[%s] %s %d %s", error in=w358, w363, w362, w361, w360) -> (resulting string=w355:string, error out=w356:errorcluster)  [unwired: 1 in]
        n99 = Write to Text File(file (use dialog)=w357, text=w355, error in=w356) -> (refnum out=w353:refnum<file>, error out=w354:errorcluster)  [unwired: 1 in, 1 out]
        n100 = call <vilib>:"Add State(s) to Queue__JKI_lib_State_Machine.vi"("State(s) in Front (\"\")"="API: Notify Controller", "State(s) in (\"\")"=w352) -> ("States Out"=w351:string)  [unwired: 13 in]
      }
      frame "API: Notify Controller" {
        # "通知Controller停止"
        # "Deal with the parameter if any"
        # "Connect this to return the response of your API"
        # "Copy/Rename this case for your own API"
        n101 = disable-structure shown="Disabled" {
          disable-tunnel: w377 -> [w382 _]
          disable-tunnel: [errorcluster {"status"=FALSE, "code"=0, "source"=""} ("error constant") errorcluster {"status"=FALSE, "code"=0, "source"=""} ("error constant")] -> w376
          frame Disabled {
            # "此API为Controller模块的API"
            # "If you need to tell who triggered this state , use this string. If it's this case itself, this string is \"\"."
            n102 = call <userlib>:"JKISM++ Post Message.vi"("Error In (no error)"=w382, "Dest Module"="Controller", "States"="API: Exit -> Controller") -> ()  [unwired: 8 in, 1 out]
          }
          frame Enabled {
          }
        }
        n103 = call <vilib>:"Add State(s) to Queue__JKI_lib_State_Machine.vi"("State(s) in Front (\"\")"="Macro: Exit", "State(s) in (\"\")"=w374) -> ("States Out"=w373:string)  [unwired: 13 in]
      }
      frame "---------- FileOperation ----------" {
        # "Template Separator\n(You can make a copy of, or modify, this frame)"
        n104 = call <vilib>:"Add State(s) to Queue__JKI_lib_State_Machine.vi"("State(s) in (\"\")"=w391) -> ("States Out"=w390:string)  [unwired: 14 in]
      }
      frame "FileOperation: OpenFile" {
        # "Your code here.\n(You can make a copy of, or modify, this frame)"
        n105 = Open/Create/Replace File(file path (use dialog)=path "C:/Users/yufeng/OneDrive - NI/ADG CCS AE/ATMJKI/ATM_JKI/Modules/Error Handler/ErrorLog.txt", error in=w393, operation (0:open)=T3."open or create") -> (refnum out=w394:refnum<file>, error out=w392:errorcluster)  [unwired: 3 in, 1 out]
        n106 = call <vilib>:"Add State(s) to Queue__JKI_lib_State_Machine.vi"("State(s) in (\"\")"=w400) -> ("States Out"=w399:string)  [unwired: 14 in]
      }
      frame "FileOperation: CloseFile" {
        # "Your code here.\n(You can make a copy of, or modify, this frame)"
        n107 = Close File(refnum=w405) -> (error out=w402:errorcluster)  [unwired: 1 in, 1 out]
        n108 = Merge Errors(w402, w403) -> (w401:errorcluster)
        n109 = call <vilib>:"Add State(s) to Queue__JKI_lib_State_Machine.vi"("State(s) in (\"\")"=w409) -> ("States Out"=w408:string)  [unwired: 14 in]
      }
    }
  }
